vi "vibrate_pulses.vi"() -> ()   [LabVIEW 2014]
panel:
  in  "PWM duty cycle":dbl[](array[numeric])
  in  "ISI (frames)":i32
  in  "pulse duration (frames)":i32
  in  "Trials Per Frequency / Power Combination":i32
  in  "Frequency (Hz)":dbl[](array[numeric])
  in  "Frames":i32
  in  "Transfer and Run Date Folder After Experiment":bool
  in  "SSH user name":string
  in  "SSH password":string
  in  "Wait before recording (s)":dbl
  in  "Tags":string
  in  "Start Recording":bool
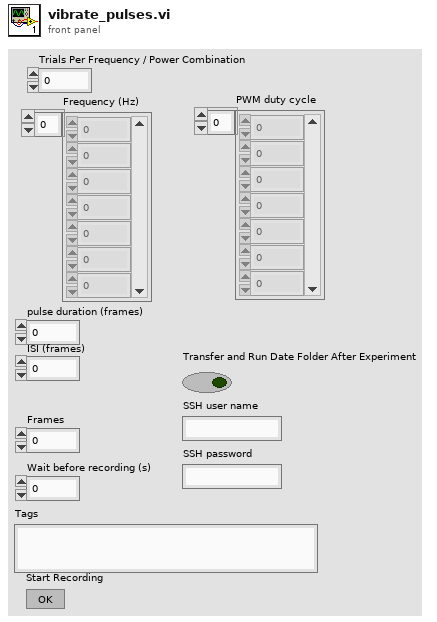
[diagram p1: front panel]
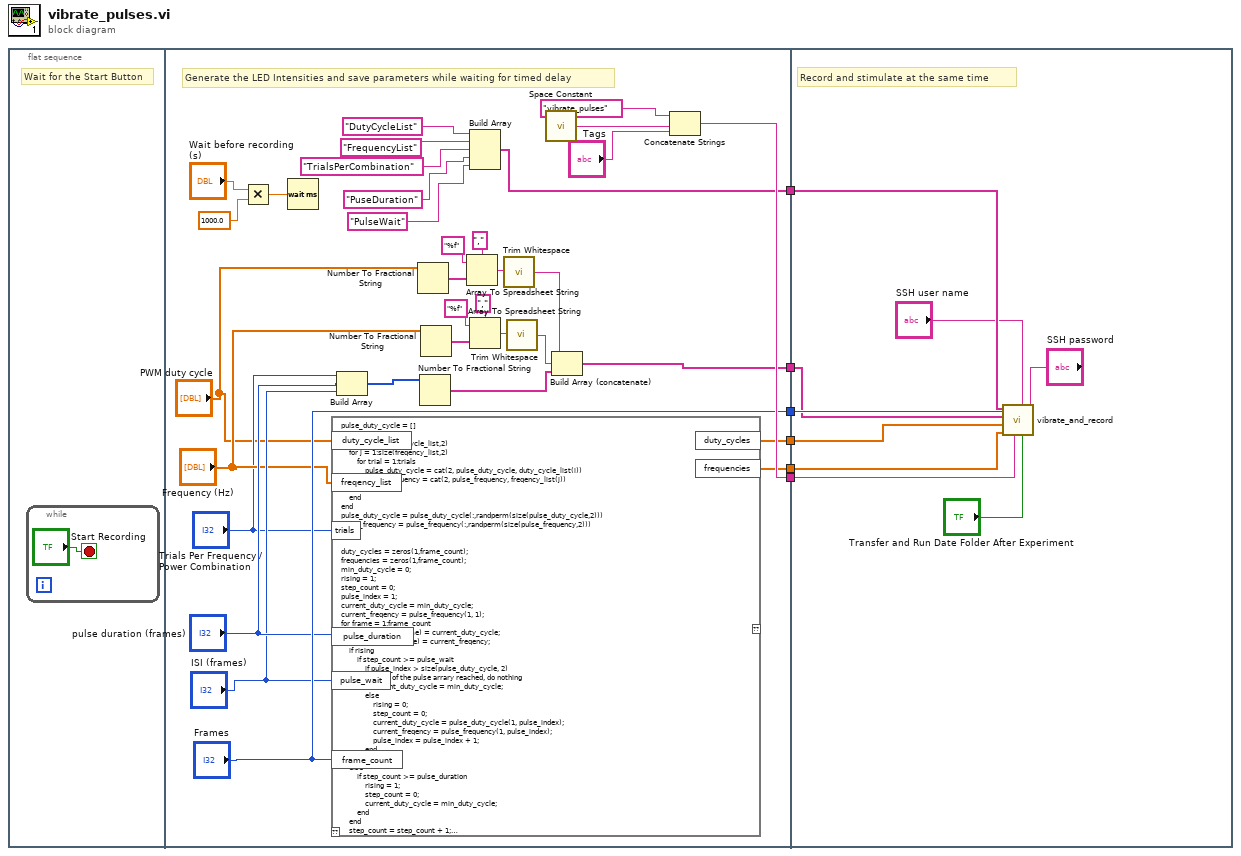
[diagram p0: block diagram]
diagram:
  n1 = flat-sequence {
    tunnel: [w38] -> w6
    tunnel: [w31] -> w5
    tunnel: [w30] -> w4
    tunnel: ["Frames"] -> w3
    tunnel: [w21] -> w2
    tunnel: [w17] -> w1
    tunnel: w6 -> [w50]
    tunnel: w5 -> [w49]
    tunnel: w4 -> [w45]
    tunnel: w3 -> [w44]
    tunnel: w2 -> [w43]
    tunnel: w1 -> [w42]
    frame #0 {
      # "Wait for the Start Button"
      n2 = while {
        stop <- "Start Recording" stop-if-true
      }
    }
    frame #1 {
      # "Generate the LED Intensities and save parameters while waiting for timed delay"
      n3 = Multiply(x="Wait before recording (s)", y=1000.0) -> (x*y=w36:dbl)
      n4 = Wait (ms)(milliseconds to wait=w36) -> ()  [unwired: 1 out]
      n5 = script code="pulse_duty_cycle = []\npulse_frequency = []\nfor i = 1:size(duty_cycle_list,2)\n    for j = 1:size(freqency_list,2)\n        for trial = 1:trials\n            pulse_duty_cycle = cat(2, pulse_duty_cycle, duty_cycle_list(i))\n            pulse_frequency = cat(2, pulse_frequency, freqency_list(j))\n        end\n    end\nend\npulse_duty_cycle = pulse_duty_cycle(:,randperm(size(pulse_duty_cycle,2)))\npulse_frequency = pulse_frequency(:,randperm(size(pulse_frequency,2)))\n\n\nduty_cycles = zeros(1,frame_count);\nfrequencies = zeros(1,frame_count);\nmin_duty_cycle = 0;\nrising = 1;\nstep_count = 0;\npulse_index = 1;\ncurrent_duty_cycle = min_duty_cycle;\ncurrent_freqency = pulse_frequency(1, 1);\nfor frame = 1:frame_count\n    duty_cycles(1,frame) = current_duty_cycle;\n    frequencies(1,frame) = current_freqency;\n    if rising\n        if step_count >= pulse_wait\n            if pulse_index > size(pulse_duty_cycle, 2)\n               %end of the pulse arrary reached, do nothing\n               current_duty_cycle = min_duty_cycle;\n            else\n                rising = 0;\n                step_count = 0;\n                current_duty_cycle = pulse_duty_cycle(1, pulse_index);\n                current_freqency = pulse_frequency(1, pulse_index);\n                pulse_index = pulse_index + 1;\n            end\n        end\n    else\n        if step_count >= pulse_duration\n            rising = 1;\n            step_count = 0;\n            current_duty_cycle = min_duty_cycle;\n        end\n    end\n    step_count = step_count + 1;\nend"("pulse_duration"="pulse duration (frames)", "frame_count"="Frames", "trials"="Trials Per Frequency / Power Combination", "freqency_list"="Frequency (Hz)", "pulse_wait"="ISI (frames)", "duty_cycle_list"="PWM duty cycle") -> ("duty_cycles"=w30:dbl[], "frequencies"=w17:dbl[])  [unwired: 1 in, 1 out]
      n6 = Build Array("Trials Per Frequency / Power Combination", "pulse duration (frames)", "ISI (frames)") -> (w25:i32[])
      n7 = Number To Fractional String(number="PWM duty cycle") -> (F-format string=w13:string[])  [unwired: 3 in]
      n8 = Number To Fractional String(number=w25) -> (F-format string=w22:string[])  [unwired: 3 in]
      n9 = Number To Fractional String(number="Frequency (Hz)") -> (F-format string=w24:string[])  [unwired: 3 in]
      n10 = Array To Spreadsheet String(delimiter (Tab)=",", array=w13, 3:"%f") -> (spreadsheet string=w10:string)
      n11 = Build Array("DutyCycleList", "FrequencyList", "TrialsPerCombination", "PuseDuration", "PulseWait") -> (w31:string[])
      n12 = Array To Spreadsheet String(delimiter (Tab)=",", array=w24, 3:"%f") -> (spreadsheet string=w19:string)
      n13 = call <vilib>:"Trim Whitespace.vi"("string"=w10) -> ("trimmed string"=w9:string)  [unwired: 1 in]
      n14 = call <vilib>:"Trim Whitespace.vi"("string"=w19) -> ("trimmed string"=w18:string)  [unwired: 1 in]
      n15 = call <vilib>:"Space Constant.vi"() -> ("String"=w40:string)
      n16 = Build Array (concatenate)(w9, w18, w22) -> (w21:string[])
      n17 = Concatenate Strings("vibrate_pulses", w40, "Tags") -> (w38:string)
    }
    frame #2 {
      # "Record and stimulate at the same time"
      n18 = call "vibrate_and_record.vi"("SSH password"="SSH password", "Transfer and Run Date Folder After Experiment"="Transfer and Run Date Folder After Experiment", "SSH user name"="SSH user name", "Tags"=w50, "Frames"=w44, "frequencies"=w42, "PWM duty cycles"=w45, "parameters"=w43, "parameters headers"=w49) -> ()  [unwired: 3 in]
    }
  }
